vi "extractLimitSwitchData.vi"(8 "error in (no error)":errorcluster, 11 "ILC in":refnum<class "ILC.lvclass">) -> (0 "error out":errorcluster, 3 "ILC out":refnum<class "ILC.lvclass">)   [LabVIEW 2013, in "ILCCommon.lvlib" / "ILC.lvclass"]
uses:
  <userlib>/Common/ILC/ILC/ILC.lvclass
  <userlib>/Common/ILC/ILCModelTypedefs/FinalDelimiter.ctl
  <userlib>/Common/ILC/ILC/ILC.lvclass/ILC.ctl
  <userlib>/Common/ILC/ILCModelTypedefs/ILCModelTypedefs.lvlib
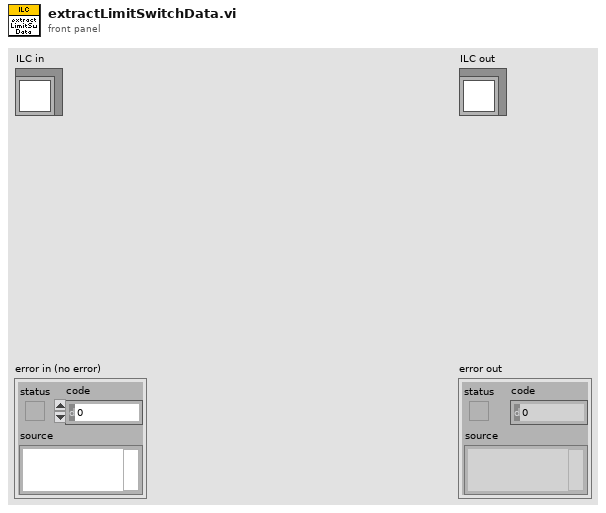
[diagram p1: front panel]
types:
  T1 = typedef "ILCCommon.lvlib/ILCModelTypedefs.lvlib/FinalDelimiter.ctl" = enum16{",", "<CR><LF>"}
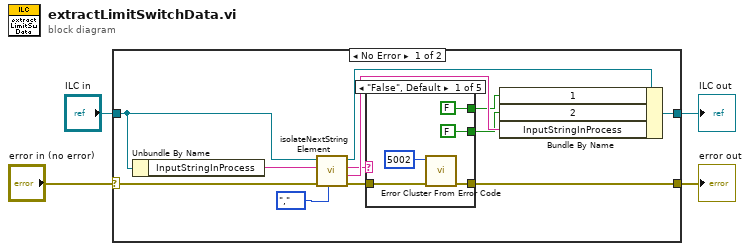
[diagram p0: block diagram]
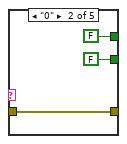
[diagram p2: hidden frame]
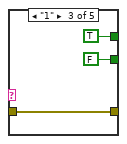
[diagram p3: hidden frame]
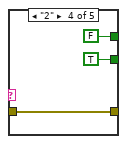
[diagram p4: hidden frame]
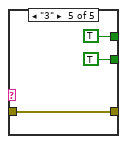
[diagram p5: hidden frame]
diagram:
  n1 = case shown="No Error" "error in (no error)" {
    selector: "error in (no error)" -> [w14 w35]
    tunnel: [w5 w35] -> w3
    tunnel: [w15 w34] -> w1
    tunnel: "ILC in" -> [w12 w34]
    frame No Error {
      n2 = Unbundle By Name(w12) -> ("InputStringInProcess"=w13:string)
      n3 = call <userlib>:"isolateNextStringElement.vi"("Final Delimiter"=FinalDelimiter.",", "error in (no error)"=w14, "inputString"=w13, "ILC in"=w12) -> ("error out"=w6:errorcluster, "remainingString"=w10:string, "extractedSegment"=w9:string, "ILC out"=w11:refnum<class "ILC.lvclass">)  [unwired: 4 in]
      n4 = case shown="\"False\", Default" w9 {
        tunnel: [FALSE FALSE TRUE FALSE TRUE] -> w8
        tunnel: [FALSE FALSE FALSE TRUE TRUE] -> w7
        tunnel: w6 -> [w18 w22 w25 w28 w31]
        tunnel: [w17 w22 w25 w28 w31] -> w5
        frame "False", Default {
          n5 = call <vilib>:"Error Cluster From Error Code.vi"("error in (no error)"=w18, "error code (0)"=5002) -> ("error out"=w17:errorcluster)  [unwired: 7 in]
        }
        frame "0" {
        }
        frame "1" {
        }
        frame "2" {
        }
        frame "3" {
        }
      }
      n6 = Bundle By Name(cluster=w11, "1"=w8, "2"=w7, "InputStringInProcess"=w10) -> (w15:refnum<class "ILC.lvclass">)
    }
    frame Error {
    }
  }
  "error out" <- w3
  "ILC out" <- w1
